vi "Configure Modulation (Amplitude).vi"(4 "Modulation Depth (0 %)":dbl, 6 "Modulation Frequency (1000 Hz)":dbl=1000.0, 7 "Enable Amplitude Modulation (T:Enable)":bool=TRUE, 8 "error in (no error)":errorcluster, 9 "Modulation Waveform (0: Sine)":u16(ring) items=["Sine", "Square", "Triangle"], 10 "AM Source (0: Internal)":u16(ring) items=["Internal", "External"], 11 "VISA resource name":refnum<visa-resource-name>) -> (0 "error out":errorcluster, 3 "VISA resource name out":refnum<visa-resource-name>)   [LabVIEW 2011, in "Template - Function Generator.lvlib"]
doc: "Configures and enables amplitude modulation (AM). In AM, the amplitude of the carrier is varied by the amplitude of the modulating waveform. \n\n<B>Note:</B> The carrier waveform shape and parameters are set by the Configure Standard Waveform VI."
uses:
  <instrlib>/_Template - Function Generator/Template - Function Generator.lvlib
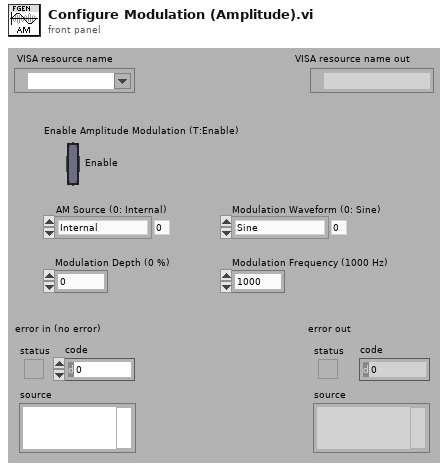
[diagram p1: front panel]
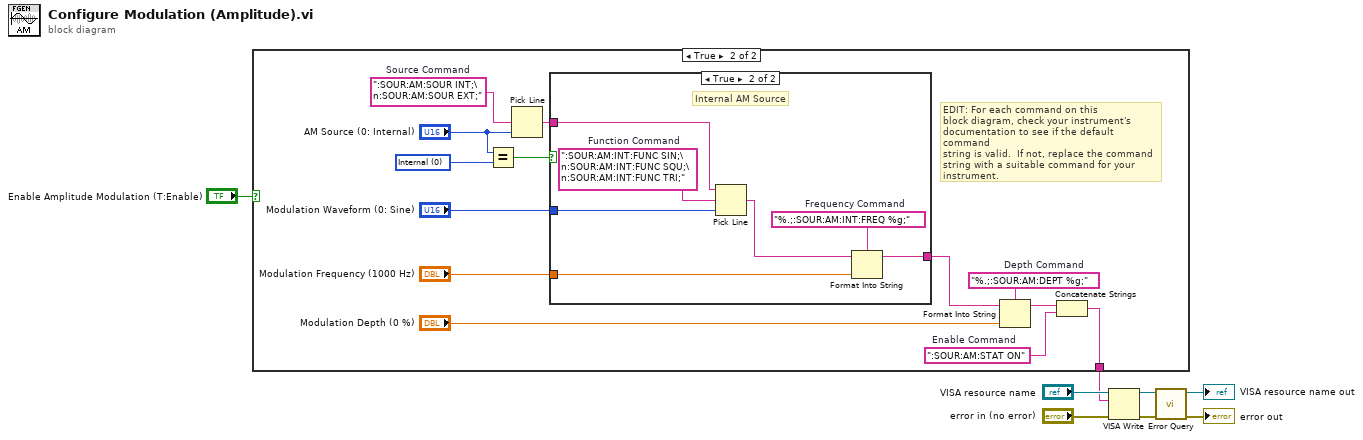
[diagram p0: block diagram]
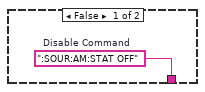
[diagram p2: hidden frame]
diagram:
  n1 = case shown="True" "Enable Amplitude Modulation (T:Enable)" {
    tunnel: [w9 w11] -> w2
    frame False {
      w9 = ":SOUR:AM:STAT OFF"  # Disable Command
    }
    frame True {
      w10 = ":SOUR:AM:STAT ON"  # Enable Command
      w15 = "%.;:SOUR:AM:DEPT %g;"  # Depth Command
      w17 = u16 0 items=["Internal", "External"] ("Source (0: Internal)")
      w18 = ":SOUR:AM:SOUR INT;\n:SOUR:AM:SOUR EXT;"  # Source Command
      # "EDIT: For each command on this\nblock diagram, check your instrument's\ndocumentation to see if the default command\nstring is valid.  If not, replace the command\nstring with a suitable command for your\ninstrument."
      n2 = Equal?(x="AM Source (0: Internal)", y=w17) -> (x = y?=w16:bool)
      n3 = Pick Line(multi-line string=w18, line index="AM Source (0: Internal)") -> (output string=w13:string)  [unwired: 1 in]
      n4 = case shown="True" w16 {
        tunnel: w13 -> [w23 w29]
        tunnel: "Modulation Waveform (0: Sine)" -> [_ w28]
        tunnel: "Modulation Frequency (1000 Hz)" -> [_ w25]
        tunnel: [w23 w24] -> w14
        frame False {
          # "External AM Source"
          # "EDIT: If external modulation is configurable,\ncall the external modulation command."
        }
        frame True {
          w27 = "%.;:SOUR:AM:INT:FREQ %g;"  # Frequency Command
          w30 = ":SOUR:AM:INT:FUNC SIN;\n:SOUR:AM:INT:FUNC SQU;\n:SOUR:AM:INT:FUNC TRI;"  # Function Command
          # "Internal AM Source"
          n5 = Pick Line(string ("")=w29, multi-line string=w30, line index=w28) -> (output string=w26:string)
          n6 = Format Into String(format string=w27, initial string=w26, w25) -> (resulting string=w24:string)  [unwired: 1 in, 1 out]
        }
      }
      n7 = Format Into String(format string=w15, initial string=w14, "Modulation Depth (0 %)") -> (resulting string=w12:string)  [unwired: 1 in, 1 out]
      n8 = Concatenate Strings(w12, w10) -> (w11:string)
    }
  }
  n9 = VISA Write(VISA resource name="VISA resource name", write buffer=w2, error in (no error)="error in (no error)") -> (VISA resource name out=w4:refnum<visa-resource-name>, error out=w3:errorcluster)  [unwired: 1 out]
  n10 = call <instrlib>:"Error Query.vi"("error in (no error)"=w3, "VISA resource name"=w4) -> ("error out"=→"error out":errorcluster, "VISA resource name out"=→"VISA resource name out":refnum<visa-resource-name>)  [unwired: 6 in, 2 out]
